vi "configure restart dynamic.vi"() -> ()   [LabVIEW 2011]
uses:
  server/server lib/Spartan CONFIG Global.vi
panel:
  in  "rendezvous":T1
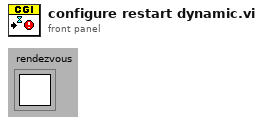
[diagram p1: front panel]
types:
  T1 = typedef "Rendezvous RefNum" = refnum<k1>
  T2 = typedef "Keyed Array.ctl" = cluster{"keys":string[], "values":string[]}
  T3 = enum32{"invalid app kind", "Development System", "Run Time System", "Student Edition", "Embedded LabVIEW", "Evaluation", "Custom"}
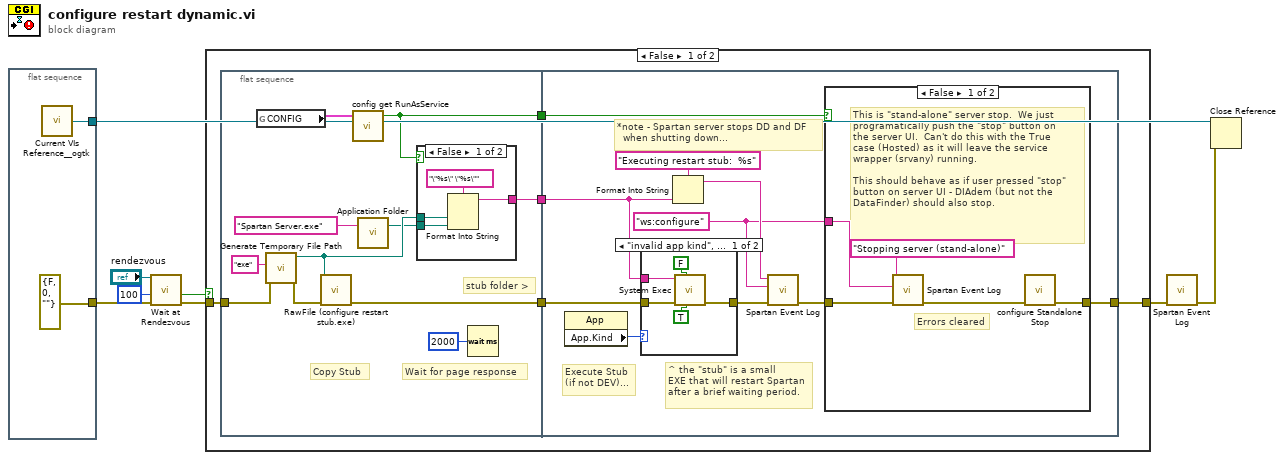
[diagram p0: block diagram]
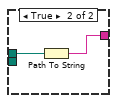
[diagram p2: hidden frame]
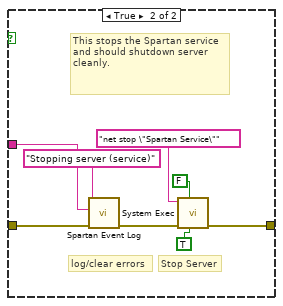
[diagram p4: hidden frame]
diagram:
  n1 = flat-sequence {
    tunnel: [w9] -> w3
    tunnel: [errorcluster {"status"=FALSE, "code"=0, "source"=""} ("error in (no error)")] -> w4
    frame #0 {
      n2 = call "Current VIs Reference__ogtk.vi"() -> ("Current VI's reference"=w9:refnum<vi>)  [unwired: 5 out]
    }
  }
  n3 = call <vilib>:"Wait at Rendezvous.vi"("error in (no error)"=w4, "ms timeout (-1)"=100, "rendezvous"="rendezvous") -> ("error out"=w6:errorcluster, "timed out"=w5:bool)  [unwired: 3 out]
  n4 = case shown="False" w5 {
    tunnel: [w15 w62] -> w2
    tunnel: w6 -> [w11 w62]
    frame False {
      n5 = flat-sequence {
        tunnel: [w22] -> w14
        tunnel: [w21] -> w13
        tunnel: [w23] -> w12
        tunnel: w11 -> [w19]
        tunnel: [w42] -> w15
        tunnel: w14 -> [w33]
        tunnel: w13 -> [w41]
        tunnel: w12 -> [w38]
        frame #0 {
          # "stub folder >"
          # "Wait for page response"
          # "Copy Stub"
          n6 = global read "Spartan CONFIG Global.vi" "CONFIG"() -> (w16:T2)
          n7 = call <vilib>:"Generate Temporary File Path.vi"("error in (no error)"=w19, "Temporary File Extension (tmp)"="exe") -> ("error out"=w26:errorcluster, "Unique Temporary File Path"=w20:path)  [unwired: 8 out]
          n8 = call "RawFile (configure restart stub.exe).vi"("error in (no error)"=w26, "Path to File (empty)"=w20) -> ("error out"=w22:errorcluster)  [unwired: 9 out]
          n9 = call "config get RunAsService.vi"("Config Keys"=w16) -> ("RunAsService?"=w21:bool)  [unwired: 4 out]
          n10 = call "Application Folder.vi"("Relative Path (\"\" - Folder)"="Spartan Server.exe" ("command line")) -> ("Application Folder"=w17:path)  [unwired: 2 in]
          n11 = case shown="False" w21 {
            tunnel: [w29 w31] -> w23
            tunnel: w20 -> [w28 w32]
            tunnel: w17 -> [w27 _]
            frame False {
              n12 = Format Into String(format string="\"%s\" \"%s\"", w28, w27) -> (resulting string=w29:string)  [unwired: 2 in, 1 out]
            }
            frame True {
              n13 = Path To String(path=w32) -> (string=w31:string)
            }
          }
          n14 = Wait (ms)(milliseconds to wait=u32 2000) -> ()  [unwired: 1 out]
        }
        frame #1 {
          w36 = "ws:configure" ("command line")
          # "*note - Spartan server stops DD and DF\n  when shutting down..."
          # "^ the \"stub\" is a small\nEXE that will restart Spartan\nafter a brief waiting period."
          # "Execute Stub\n(if not DEV)..."
          n15 = property class="App"() -> ("App.Kind"=w37:T3)  [unwired: 2 in, 2 out]
          n16 = case shown="\"invalid app kind\", Default" w37 {
            tunnel: w33 -> [w45 w48]
            tunnel: [w44 w48] -> w35
            tunnel: w38 -> [w43 _]
            frame "invalid app kind", Default {
              n17 = call <vilib>:"System Exec.vi"("run minimized? (F)"=TRUE, "wait until completion? (T)"=FALSE, "error in (no error)"=w45, "command line"=w43) -> ("error out"=w44:errorcluster)  [unwired: 2 in, 5 out]
            }
            frame "Development System" {
            }
          }
          n18 = Format Into String(format string="Executing restart stub:  %s", w38) -> (resulting string=w39:string)  [unwired: 2 in, 1 out]
          n19 = call "Spartan Event Log.vi"("error in (no error)"=w35, "module (\"\")"=w36, "message (\"\")"=w39) -> ("error out"=w34:errorcluster)  [unwired: 2 in, 3 out]
          n20 = case shown="False" w41 {
            tunnel: w34 -> [w53 w54]
            tunnel: [w49 w59] -> w42
            tunnel: w36 -> [w52 w55]
            frame False {
              # "Errors cleared"
              # "This is \"stand-alone\" server stop.  We just\nprogramatically push the \"stop\" button on\nthe server UI.  Can't do this with the True\ncase (Hosted) as it will leave the service\nwrapper (srvany) running.\n\nThis should behave as if user pressed \"stop\"\nbutton on server UI - DIAdem (but not the\nDataFinder) should also stop."
              n21 = call "Spartan Event Log.vi"("error in (no error)"=w53, "module (\"\")"=w52, "message (\"\")"="Stopping server (stand-alone)") -> ("error out"=w50:errorcluster)  [unwired: 2 in, 3 out]
              n22 = call "configure Standalone Stop.vi"("error in (no error)"=w50) -> ("error out"=w49:errorcluster)  [unwired: 6 out]
            }
            frame True {
              # "This stops the Spartan service\nand should shutdown server\ncleanly."
              # "Stop Server"
              # "log/clear errors"
              n23 = call "Spartan Event Log.vi"("error in (no error)"=w54, "module (\"\")"=w55, "message (\"\")"="Stopping server (service)") -> ("error out"=w57:errorcluster)  [unwired: 2 in, 3 out]
              n24 = call <vilib>:"System Exec.vi"("run minimized? (F)"=TRUE, "wait until completion? (T)"=FALSE, "error in (no error)"=w57, "command line"="net stop \"Spartan Service\"") -> ("error out"=w59:errorcluster)  [unwired: 2 in, 5 out]
            }
          }
        }
      }
    }
    frame True {
    }
  }
  n25 = call "Spartan Event Log.vi"("error in (no error)"=w2) -> ("error out"=w1:errorcluster)  [unwired: 4 in, 3 out]
  n26 = Close Reference(reference=w3, error in (no error)=w1) -> ()  [unwired: 1 out]
